vi "define boundary points for specified  ROI.vi"() -> ()   [LabVIEW 2010]
panel:
  out "output array":cluster{"x":i32, "y":i32}[](array[cluster])
  out "Array 4":cluster{"x":i32, "y":i32}[](array[cluster])
  out "Array 3":cluster{"x":i32, "y":i32}[](array[cluster])
  out "Array 2":cluster{"x":i32, "y":i32}[](array[cluster])
  out "Array":cluster{"x":i32, "y":i32}[](array[cluster])
  in  "centroid:Yc":i32
  in  "centroid: Xc":i32
  in  "width":i32(slide) scale=0.0..10.0
  in  "length":i32(slide) scale=0.0..10.0
  out "ymax":i32
  out "ymin":i32
  out "xmax":i32
  out "xmin":i32
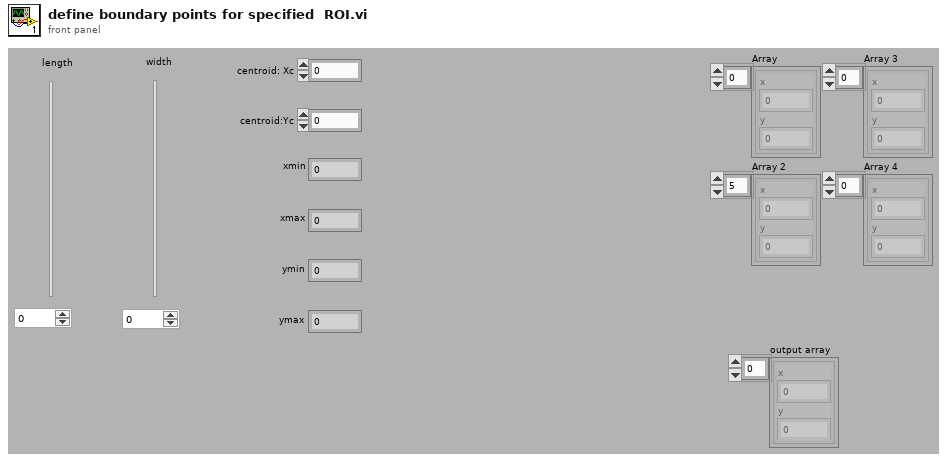
[diagram p1: front panel]
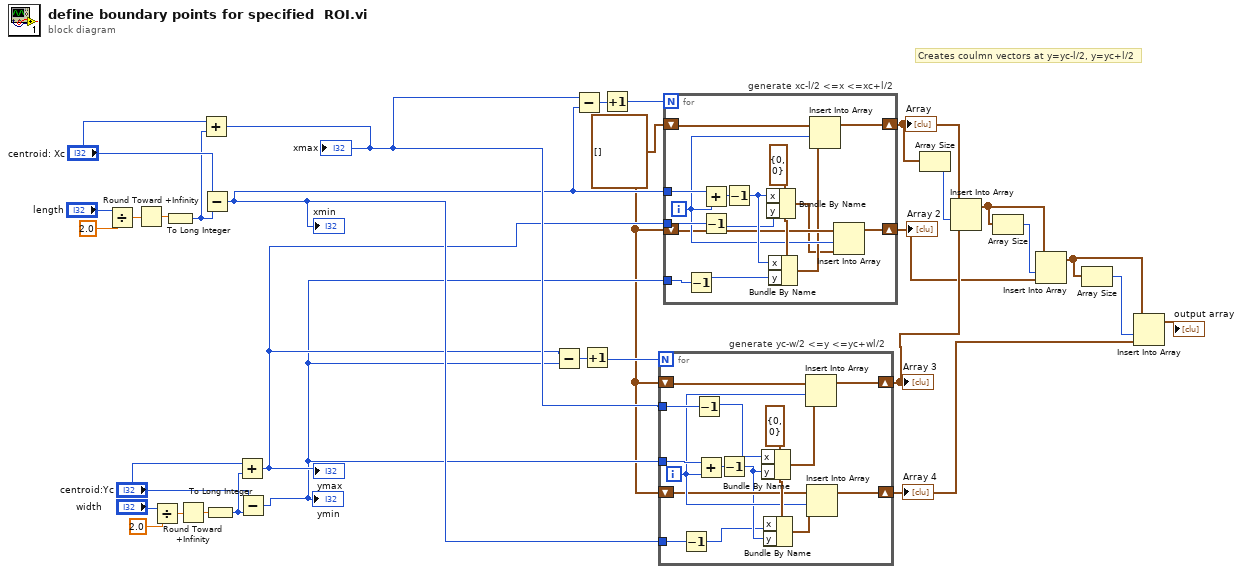
[diagram p0: block diagram]
diagram:
  w11 = cluster{"x":i32, "y":i32}[] []
  # "Creates coulmn vectors at y=yc-l/2, y=yc+l/2"
  n1 = Divide(x="length", y=2.0) -> (x/y=w27:dbl)
  n2 = Round Toward +Infinity(x=w27) -> (ceil(x): smallest int >= x=w26:dbl)
  n3 = Divide(x="width", y=2.0) -> (x/y=w22:dbl)
  n4 = To Long Integer(number=w26) -> (32bit integer=w24:i32)
  n5 = Round Toward +Infinity(x=w22) -> (ceil(x): smallest int >= x=w23:dbl)
  n6 = Add(x="centroid: Xc", y=w24) -> (x+y=w17:i32)
  "xmax" <- w17
  n7 = Subtract(x="centroid: Xc", y=w24) -> (x-y=w16:i32)
  "xmin" <- w16
  n8 = To Long Integer(number=w23) -> (32bit integer=w19:i32)
  n9 = Add(x="centroid:Yc", y=w19) -> (x+y=w13:i32)
  "ymax" <- w13
  n10 = Subtract(x="centroid:Yc", y=w19) -> (x-y=w12:i32)
  "ymin" <- w12
  n11 = Subtract(x=w13, y=w12) -> (x-y=w15:i32)
  n12 = Subtract(x=w17, y=w16) -> (x-y=w31:i32)
  n13 = Increment(x=w15) -> (x+1=w14:i32)
  n14 = Increment(x=w31) -> (x+1=w30:i32)
  n15 = for "generate yc-w/2 <=y <=yc+wl/2" {
    N: w14 -> [_]
    tunnel: w12 -> [w46]
    tunnel: w17 -> [w44]
    tunnel: w16 -> [w43]
    shift-right: [w37] -> w2
    shift-left: w11 -> [w40]
    shift-right: [w36] -> w6
    shift-left: w11 -> [w35]
    i -> [w39]
    w41 = cluster{"x":i32, "y":i32} {"x"=0, "y"=0}
    n16 = Decrement(x=w43) -> (x-1=w32:i32)
    n17 = Decrement(x=w44) -> (x-1=w34:i32)
    n18 = Add(x=w46, y=w39) -> (x+y=w45:i32)
    n19 = Decrement(x=w45) -> (x-1=w33:i32)
    n20 = Bundle By Name(cluster=w41, "x"=w34, "y"=w33) -> (w42:cluster{"x":i32, "y":i32})
    n21 = Bundle By Name(cluster=w41, "x"=w32, "y"=w33) -> (w38:cluster{"x":i32, "y":i32})
    n22 = Insert Into Array(array=w40, index=w39, new element=w42) -> (w37:cluster{"x":i32, "y":i32}[])
    n23 = Insert Into Array(array=w35, index=w39, new element=w38) -> (w36:cluster{"x":i32, "y":i32}[])
  }
  "Array 3" <- w2
  "Array 4" <- w6
  n24 = for "generate xc-l/2 <=x <=xc+l/2" {
    N: w30 -> [_]
    tunnel: w16 -> [w61]
    tunnel: w13 -> [w58]
    tunnel: w12 -> [w56]
    shift-right: [w51] -> w10
    shift-left: w11 -> [w53]
    shift-right: [w50] -> w1
    shift-left: w11 -> [w49]
    i -> [w52]
    w54 = cluster{"x":i32, "y":i32} {"x"=0, "y"=0}
    n25 = Decrement(x=w56) -> (x-1=w55:i32)
    n26 = Add(x=w61, y=w52) -> (x+y=w60:i32)
    n27 = Decrement(x=w58) -> (x-1=w57:i32)
    n28 = Decrement(x=w60) -> (x-1=w59:i32)
    n29 = Bundle By Name(cluster=w54, "x"=w59, "y"=w57) -> (w47:cluster{"x":i32, "y":i32})
    n30 = Bundle By Name(cluster=w54, "x"=w59, "y"=w55) -> (w48:cluster{"x":i32, "y":i32})
    n31 = Insert Into Array(array=w53, index=w52, new element=w48) -> (w51:cluster{"x":i32, "y":i32}[])
    n32 = Insert Into Array(array=w49, index=w52, new element=w47) -> (w50:cluster{"x":i32, "y":i32}[])
  }
  "Array" <- w10
  "Array 2" <- w1
  n33 = Array Size(array=w10) -> (size(s)=w9:i32)
  n34 = Insert Into Array(array=w10, index=w9, new element=w2) -> (w8:cluster{"x":i32, "y":i32}[])
  n35 = Array Size(array=w8) -> (size(s)=w7:i32)
  n36 = Insert Into Array(array=w8, index=w7, new element=w1) -> (w5:cluster{"x":i32, "y":i32}[])
  n37 = Array Size(array=w5) -> (size(s)=w4:i32)
  n38 = Insert Into Array(array=w5, index=w4, new element=w6) -> (→"output array":cluster{"x":i32, "y":i32}[])
